vi "Termometr0-2.vi"(1 "Numeric":dbl) -> (0 "Град":dbl)   [LabVIEW 2020]
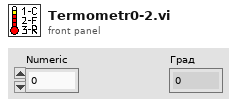
[diagram p1: front panel]
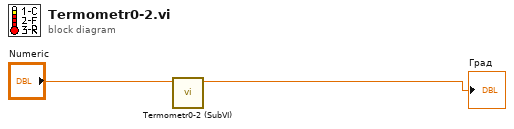
[diagram p0: block diagram]
diagram:
  n1 = call "Termometr0-2 (SubVI).vi"("Numeric"="Numeric") -> ("Град"=→"Град":dbl)  [unwired: 10 in]
